vi "Configure IQ.vi"(0 "VISA resource name":refnum<visa-resource-name>, 1 "I/Q Trigger Source (0: Internal)":u16(ring) items=["Internal", "External", "Manual"], 2 "Gain Balance(0 dB)":dbl, 3 "Q Channel Offset Value (0 V)":dbl, 5 "Center Frequency (0 Hz)":dbl, 7 "Symbol Rate (250 kSymbo/s)":dbl=250000.0, 9 "I/Q Amplitude (0.1414 Vrms)":dbl=0.1414, 11 "error in (no error)":errorcluster, 12 "I/Q Data (2ASK)":u16(ring) items=["2ASK", "4ASK", "8ASK", "BPSK", "QPSK", "8PSK", "DBPSK", "DQPSK", "D8PSK", "8QAM", "16QAM", "32QAM", "64QAM", "128QAM", "256QAM"], 13 "I Channel Offset Value (0 V)":dbl, 14 "Quadrature Skew (0 deg)":dbl) -> (4 "VISA resource name out":refnum<visa-resource-name>, 15 "error out":errorcluster)   [LabVIEW 2023, in "Siglent SDG X Series.lvlib"]
doc: "Configures I/Q modulation and parameters.\n\nNote:\nThis VI only supports SDG6000X series."
uses:
  Siglent SDG X Series.lvlib
panel:
  in  "Channel (1:Channel 1)":i32(ring)=1 items=["Channel 1"=1]
  # "I/Q Adjustment"
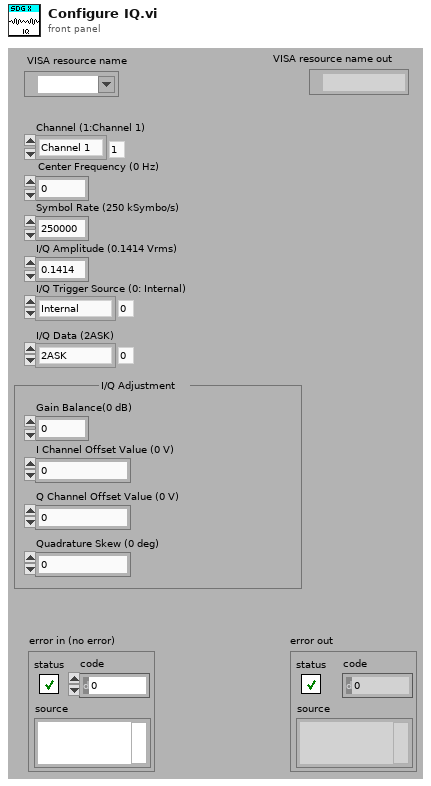
[diagram p1: front panel]
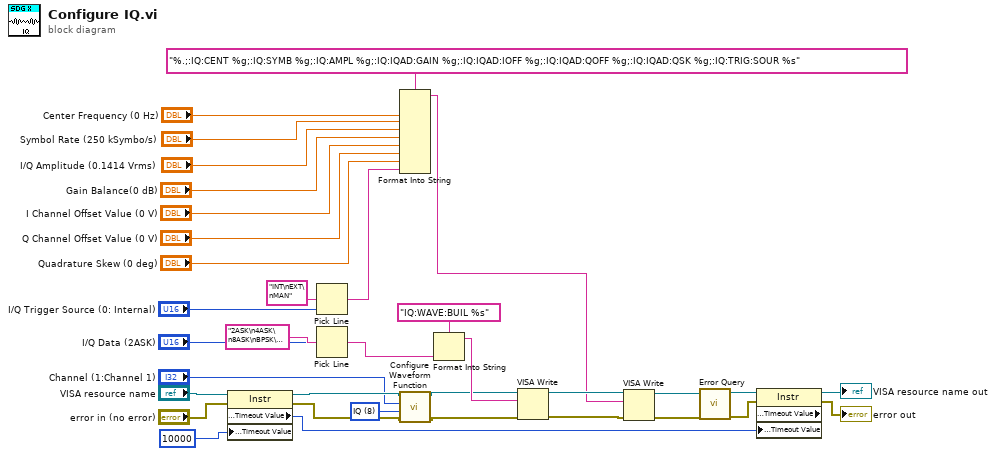
[diagram p0: block diagram]
diagram:
  w2 = u16 8 items=["Sine", "Square", "Ramp", "DC", "Pulse", "Arb", "Noise", "PRBS", "IQ"] ("Waveform Function (0: Sine)")
  n1 = property on="Property Node" class="Instr"(reference="VISA resource name", error in="error in (no error)", "General Settings:Timeout Value"=u32 10000) -> (reference out=w4:refnum<visa-resource-name>, error out=w3:errorcluster, "General Settings:Timeout Value"=w8:u32)
  n2 = Pick Line(multi-line string="INT\nEXT\nMAN" ("多行字符串"), line index="I/Q Trigger Source (0: Internal)") -> (output string=w18:string)  [unwired: 1 in]
  n3 = Pick Line(multi-line string="2ASK\n4ASK\n8ASK\nBPSK\nQPSK\n8PSK\nDBPSK\nDQPSK\nD8PSK\n8QAM\n16QAM\n32QAM\n64QAM\n128QAM\n256QAM" ("多行字符串"), line index="I/Q Data (2ASK)") -> (output string=w30:string)  [unwired: 1 in]
  n4 = Format Into String(format string="%.;:IQ:CENT %g;:IQ:SYMB %g;:IQ:AMPL %g;:IQ:IQAD:GAIN %g;:IQ:IQAD:IOFF %g;:IQ:IQAD:QOFF %g;:IQ:IQAD:QSK %g;:IQ:TRIG:SOUR %s" ("格式字符串"), "Center Frequency (0 Hz)", "Symbol Rate (250 kSymbo/s)", "I/Q Amplitude (0.1414 Vrms)", "Gain Balance(0 dB)", "I Channel Offset Value (0 V)", "Q Channel Offset Value (0 V)", "Quadrature Skew (0 deg)", w18) -> (resulting string=w26:string)  [unwired: 2 in, 1 out]
  n5 = call "Configure Waveform Function.vi"("error in (no error)"=w3, "Waveform Function (0: Sine)"=w2, "Channel (1:Channel 1)"="Channel (1:Channel 1)", "VISA resource name"=w4) -> ("error out"=w5:errorcluster, "VISA resource name out"=w6:refnum<visa-resource-name>)  [unwired: 6 in]
  n6 = Format Into String(format string="IQ:WAVE:BUIL %s" ("初始字符串"), w30) -> (resulting string=w29:string)  [unwired: 2 in, 1 out]
  n7 = VISA Write(VISA resource name=w6, write buffer=w29, error in (no error)=w5) -> (VISA resource name out=w28:refnum<visa-resource-name>, error out=w27:errorcluster)  [unwired: 1 out]
  n8 = VISA Write(VISA resource name=w28, write buffer=w26, error in (no error)=w27) -> (VISA resource name out=w16:refnum<visa-resource-name>, error out=w15:errorcluster)  [unwired: 1 out]
  n9 = call "Error Query.vi"("error in (no error)"=w15, "VISA resource name"=w16) -> ("error out"=w11:errorcluster, "VISA resource name out"=w12:refnum<visa-resource-name>)  [unwired: 6 in, 2 out]
  n10 = property on="Property Node" class="Instr" props=["General Settings:Timeout Value", "General Settings:Timeout Value"](reference=w12, error in=w11, "General Settings:Timeout Value"=w8) -> (reference out=→"VISA resource name out":refnum<visa-resource-name>, error out=→"error out":errorcluster)  [unwired: 1 out]
